vi "user mapped buttons.vi"(8 "previous button state":u32, 9 "gp button info":T1, 11 "map references":T2) -> (0 "current button state":u32, 1 "gp button info 2":T1)   [LabVIEW 2012]
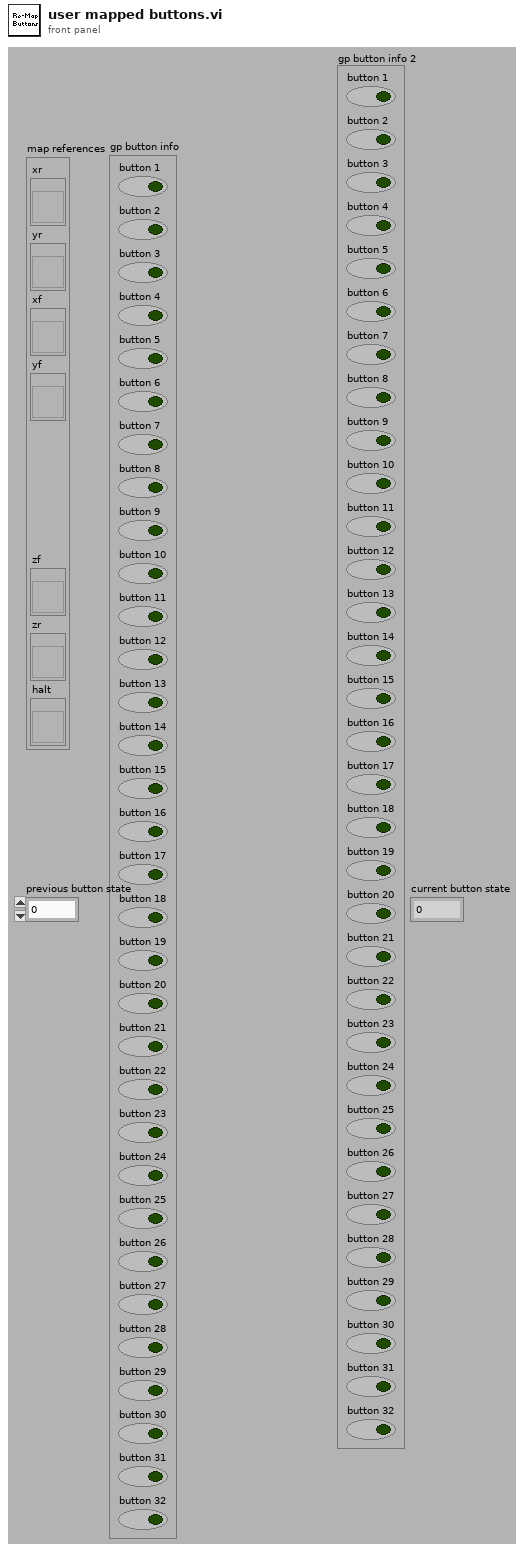
[diagram p1: front panel]
types:
  T1 = cluster{"button 1":bool, "button 2":bool, "button 3":bool, "button 4":bool, "button 5":bool, "button 6":bool, "button 7":bool, "button 8":bool, "button 9":bool, "button 10":bool, "button 11":bool, "button 12":bool, "button 13":bool, "button 14":bool, "button 15":bool, "button 16":bool, "button 17":bool, "button 18":bool, "button 19":bool, "button 20":bool, "button 21":bool, "button 22":bool, "button 23":bool, "button 24":bool, "button 25":bool, "button 26":bool, "button 27":bool, "button 28":bool, "button 29":bool, "button 30":bool, "button 31":bool, "button 32":bool}
  T2 = cluster{"xr":refnum<vi>, "yr":refnum<vi>, "xf":refnum<vi>, "yf":refnum<vi>, "zr":refnum<vi>, "zf":refnum<vi>, "halt":refnum<vi>}
  T3 = cluster{"[0]":bool, "[1]":bool, "[2]":bool, "[3]":bool, "[4]":bool, "[5]":bool, "[6]":bool, "[7]":bool, "[8]":bool}
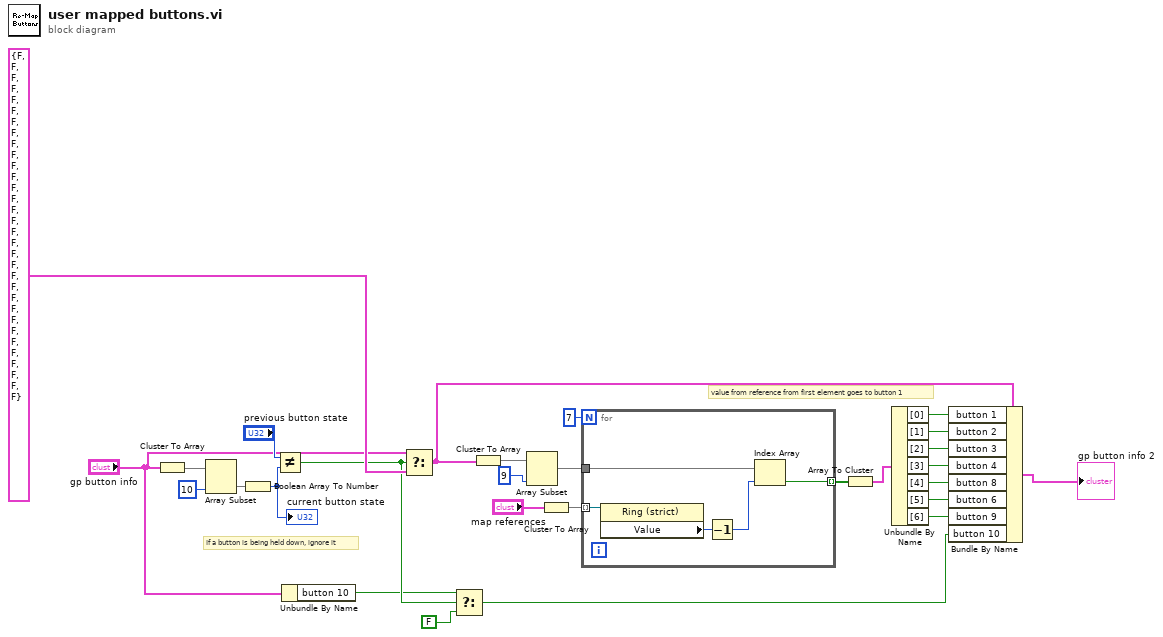
[diagram p0: block diagram]
diagram:
  # "If a button is being held down, ignore it"
  # "value from reference from first element goes to button 1"
  n1 = Cluster To Array(cluster="gp button info") -> (array=w16:bool[])
  n2 = Array Subset(array=w16, length=10) -> (w14:bool[])  [unwired: 1 in]
  n3 = Boolean Array To Number(Boolean array=w14) -> (number=w13:u32)
  "current button state" <- w13
  n4 = Not Equal?(x="previous button state", y=w13) -> (x != y?=w9:bool)
  n5 = Unbundle By Name("gp button info") -> ("button 10"=w7:bool)
  n6 = Select(t="gp button info", s=w9, f=T1 {"button 1"=FALSE, "button 2"=FALSE, "button 3"=FALSE, "button 4"=FALSE, "button 5"=FALSE, "button 6"=FALSE, "button 7"=FALSE, "button 8"=FALSE, "button 9"=FALSE, "button 10"=FALSE, "button 11"=FALSE, "button 12"=FALSE, "button 13"=FALSE, "button 14"=FALSE, "button 15"=FALSE, "button 16"=FALSE, "button 17"=FALSE, "button 18"=FALSE, "button 19"=FALSE, "button 20"=FALSE, "button 21"=FALSE, "button 22"=FALSE, "button 23"=FALSE, "button 24"=FALSE, "button 25"=FALSE, "button 26"=FALSE, "button 27"=FALSE, "button 28"=FALSE, "button 29"=FALSE, "button 30"=FALSE, "button 31"=FALSE, "button 32"=FALSE} ("button info")) -> (s? t:f=w10:T1)
  n7 = Select(t=w7, s=w9, f=FALSE ("x != y?")) -> (s? t:f=w1:bool)
  n8 = Cluster To Array(cluster=w10) -> (array=w24:bool[])
  n9 = Array Subset(array=w24, length=9) -> (w25:bool[])  [unwired: 1 in]
  n10 = Cluster To Array(cluster="map references") -> (array=w28:refnum<vi>[])
  n11 = for {
    N: 7 -> [_]
    tunnel: w28 -> [w33] mode=indexing
    tunnel: w25 -> [w32]
    tunnel: [w29] -> w26 mode=indexing
    n12 = property on="Property Node" class="Ring (strict)"(reference=w33) -> ("Value"=w31:u16)  [unwired: 1 in, 2 out]
    n13 = Decrement(x=w31) -> (x-1=w30:u16)
    n14 = Index Array(array=w32, index=w30) -> (element=w29:bool)
  }
  n15 = Array To Cluster(array=w26) -> (cluster=w21:T3)
  n16 = Unbundle By Name(w21) -> ("[0]"=w17:bool, "[1]"=w18:bool, "[2]"=w19:bool, "[3]"=w20:bool, "[4]"=w5:bool, "[5]"=w4:bool, "[6]"=w3:bool)
  n17 = Bundle By Name(cluster=w10, "button 1"=w17, "button 2"=w18, "button 3"=w19, "button 4"=w20, "button 8"=w5, "button 6"=w4, "button 9"=w3, "button 10"=w1) -> (→"gp button info 2":T1)
